vi "시리얼 연결.vi"() -> ()   [LabVIEW 2018]
uses:
  <vilib>/Instr/_visa.llb/VISA Configure Serial Port (Instr).vi
panel:
  in  "baud rate (9600)":u32=9600 caption="보 전송속도(9600)"
  out "버퍼 읽기":string
  out "에러 출력":errorcluster
  in  "VISA 리소스 이름":refnum<visa-resource-name>
  in  "명령":string
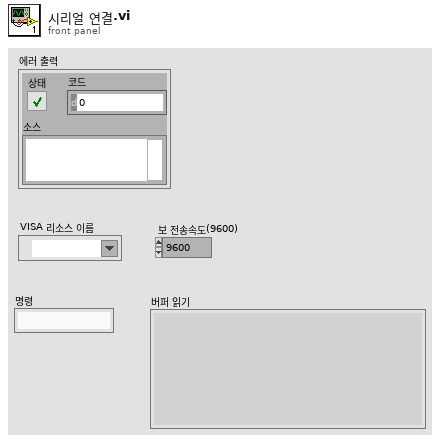
[diagram p1: front panel]
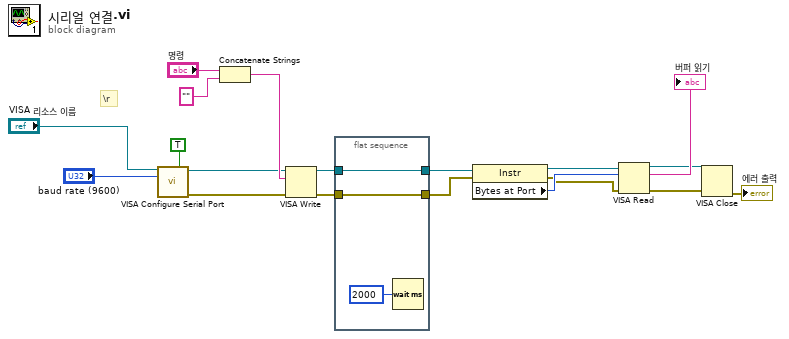
[diagram p0: block diagram]
diagram:
  # "\\r"
  n1 = call-poly "VISA Configure Serial Port"("VISA resource name"="VISA 리소스 이름", "Enable Termination\nChar (T)"=TRUE ("Enable Termination\nChar (T)"), "baud rate (9600)"="baud rate (9600)") -> ("VISA resource name out"=w14:refnum<visa-resource-name>, "error out"=w13:errorcluster)  [unwired: 11 in]
  n2 = Concatenate Strings("명령", "") -> (w16:string)
  n3 = VISA Write(VISA resource name=w14, write buffer=w16, error in (no error)=w13) -> (VISA resource name out=w12:refnum<visa-resource-name>, error out=w11:errorcluster)  [unwired: 1 out]
  n4 = flat-sequence {
    tunnel: [w21] -> w10
    tunnel: w12 -> [w21]
    tunnel: [w20] -> w9
    tunnel: w11 -> [w20]
    frame #0 {
      n5 = Wait (ms)(milliseconds to wait=u32 2000 ("대기 시간 (ms)")) -> ()  [unwired: 1 out]
    }
  }
  n6 = property class="Instr"(reference=w10, error in=w9) -> (reference out=w7:refnum<visa-resource-name>, error out=w6:errorcluster, "Bytes at Port"=w8:u32)
  n7 = VISA Read(VISA resource name=w7, byte count=w8, error in (no error)=w6) -> (VISA resource name out=w4:refnum<visa-resource-name>, read buffer=→"버퍼 읽기":string, error out=w3:errorcluster)  [unwired: 1 out]
  n8 = VISA Close(VISA resource name=w4, error in (no error)=w3) -> (error out=→"에러 출력":errorcluster)
